vi "creat Output Task.vi"(7 "Configuration":T1={"DAQmxChannel myVolt"={"DAQmxChannel myVinput1"={"PhysicalChanName"="myDAQ2/ai1", "AI_Voltage_Units"=10348, "AI_Max"=5.0, "AI_Min"=-5.0}, "DAQmxChannel myVinput2"={"PhysicalChanName"="", "AI_Voltage_Units"=10348, "AI_Max"=5.0, "AI_Min"=-5.0}, "DAQmxChannel myVoutput1"={"PhysicalChanName"="", "AI_Min"=-5.0, "AI_Max"=5.0, "AI_Voltage_Units"=10348}, "DAQmxChannel myVoutput2"={"PhysicalChanName"="", "AI_Min"=-5.0, "AI_Max"=5.0, "AI_Voltage_Units"=10348}, "Saidmple Clock Input"={"rate"=1000.0, "samples per channel"=100}, "Saidmple Clock Output"={"rate"=1000.0, "samples per channel"=100}}, "Dev"=""} {"DAQmxChannel myVolt"."DAQmxChannel myVoutput2"."AI_Voltage_Units" items=["伏特"=10348, "来自自定义换算"=10065]; "DAQmxChannel myVolt"."DAQmxChannel myVoutput1"."AI_Voltage_Units" items=["伏特"=10348, "来自自定义换算"=10065]; "DAQmxChannel myVolt"."DAQmxChannel myVinput1"."AI_Voltage_Units" items=["伏特"=10348, "来自自定义换算"=10065]; "DAQmxChannel myVolt"."DAQmxChannel myVinput2"."AI_Voltage_Units" items=["伏特"=10348, "来自自定义换算"=10065]}, 11 "Task":refnum<k21>) -> (3 "引用句柄输出":refnum<k21>)   [LabVIEW 2016]
uses:
  Contral/Coniguration.ctl
  <vilib>/DAQmx/create/channels.llb/DAQmx Create Channel (AO-Voltage-Basic).vi
  <vilib>/DAQmx/configure/timing.llb/DAQmx Timing (Sample Clock).vi
panel:
  in  "error in":errorcluster caption="错误输入"
  out "error out":errorcluster caption="错误输出"
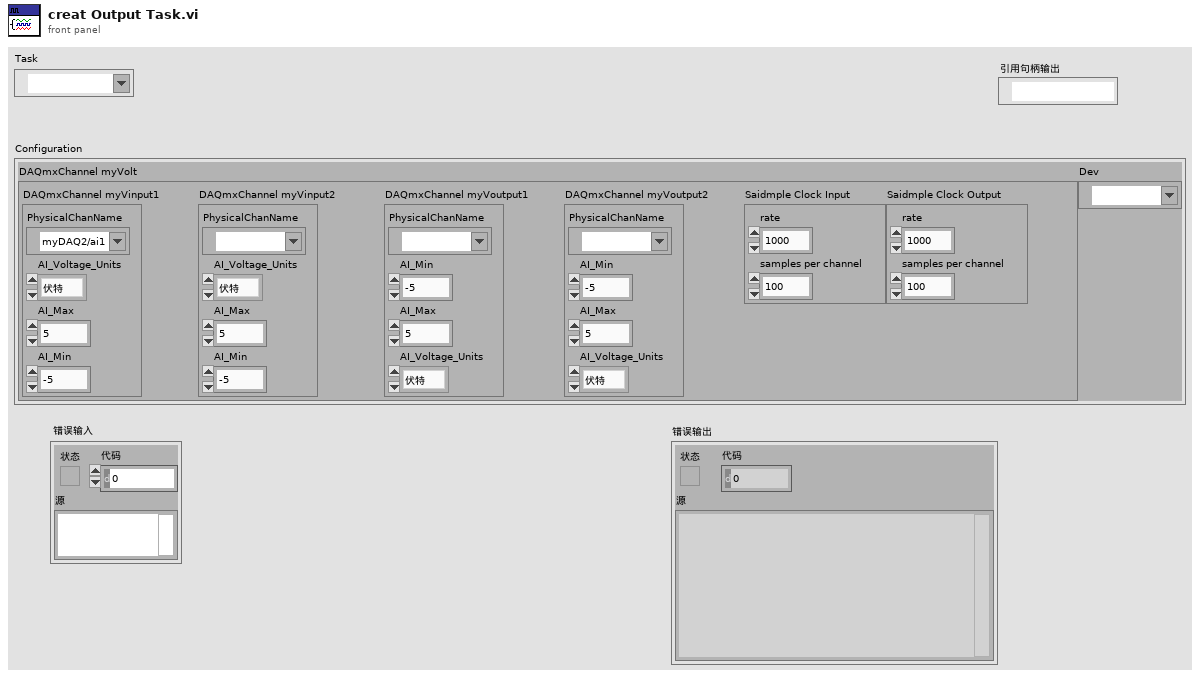
[diagram p1: front panel]
types:
  T1 = typedef "Coniguration.ctl" = cluster{"DAQmxChannel myVolt":cluster{"DAQmxChannel myVinput1":cluster{"PhysicalChanName":tag, "AI_Voltage_Units":i32, "AI_Max":dbl, "AI_Min":dbl}, "DAQmxChannel myVinput2":cluster{"PhysicalChanName":tag, "AI_Voltage_Units":i32, "AI_Max":dbl, "AI_Min":dbl}, "DAQmxChannel myVoutput1":cluster{"PhysicalChanName":tag, "AI_Min":dbl, "AI_Max":dbl, "AI_Voltage_Units":i32}, "DAQmxChannel myVoutput2":cluster{"PhysicalChanName":tag, "AI_Min":dbl, "AI_Max":dbl, "AI_Voltage_Units":i32}, "Saidmple Clock Input":cluster{"rate":dbl, "samples per channel":i32}, "Saidmple Clock Output":cluster{"rate":dbl, "samples per channel":i32}}, "Dev":tag}
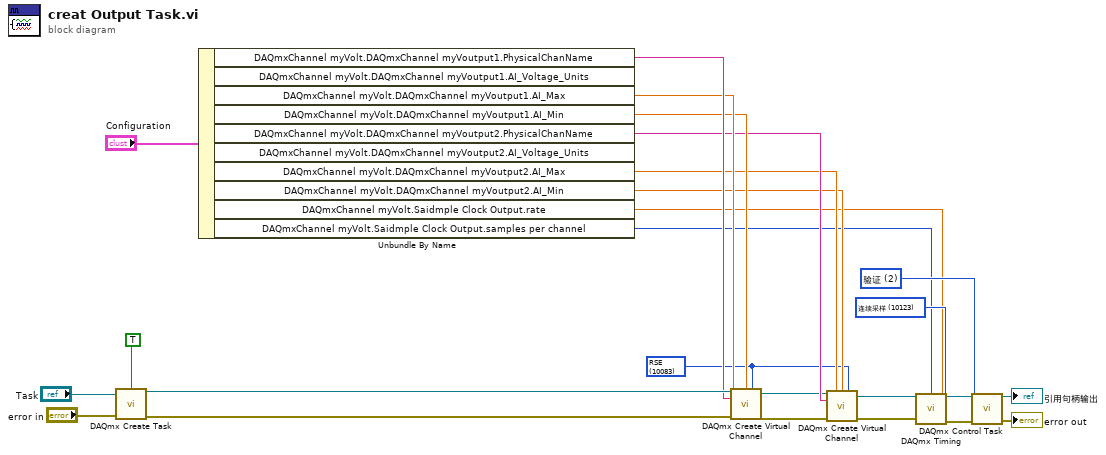
[diagram p0: block diagram]
diagram:
  w19 = 2 items=["验证"=2, "保留"=4, "提交"=3, "未保留"=5, "中止"=6] ("action")
  w22 = 10123 items=["有限采样"=10178, "连续采样"=10123, "硬件定时单点"=12522] ("sample mode")
  w7 = 10083 items=["默认"=-1, "RSE"=10083, "NRSE"=10078, "差分"=10106, "伪差分"=12529] ("input terminal configuration")
  n1 = call <vilib>:"DAQmx Create Task.vi"("auto cleanup"=TRUE, "task to copy"="Task", "error in"="error in") -> ("task out"=w23:refnum<k21>, "error out"=w25:errorcluster)  [unwired: 11 in]
  n2 = Unbundle By Name("Configuration") -> ("DAQmxChannel myVolt.DAQmxChannel myVoutput1.PhysicalChanName"=w17:tag, "DAQmxChannel myVolt.DAQmxChannel myVoutput1.AI_Max"=w16:dbl, "DAQmxChannel myVolt.DAQmxChannel myVoutput1.AI_Min"=w15:dbl, "DAQmxChannel myVolt.DAQmxChannel myVoutput2.PhysicalChanName"=w14:tag, "DAQmxChannel myVolt.DAQmxChannel myVoutput2.AI_Max"=w12:dbl, "DAQmxChannel myVolt.DAQmxChannel myVoutput2.AI_Min"=w11:dbl, "DAQmxChannel myVolt.Saidmple Clock Output.rate"=w2:dbl, "DAQmxChannel myVolt.Saidmple Clock Output.samples per channel"=w1:i32)  [unwired: 2 out]
  n3 = call-poly <vilib>:"DAQmx Create Virtual Channel.vi"("task in"=w23, "maximum value"=w16, "minimum value"=w15, "output terminal configuration"=w7, "physical channels"=w17, "error in"=w25) -> ("task out"=w13:refnum<k21>, "error out"=w10:errorcluster)  [unwired: 8 in]
  n4 = call-poly <vilib>:"DAQmx Create Virtual Channel.vi"("task in"=w13, "maximum value"=w12, "minimum value"=w11, "output terminal configuration"=w7, "physical channels"=w14, "error in"=w10) -> ("task out"=w6:refnum<k21>, "error out"=w5:errorcluster)  [unwired: 8 in]
  n5 = call-poly <vilib>:"DAQmx Timing.vi"("task/channels in"=w6, "sample mode"=w22, "samples per channel"=w1, "rate"=w2, "error in"=w5) -> ("task out"=w21:refnum<k21>, "error out"=w20:errorcluster)  [unwired: 9 in]
  n6 = call <vilib>:"DAQmx Control Task.vi"("task/channels in"=w21, "action"=w19, "error in"=w20) -> ("task out"=→"引用句柄输出":refnum<k21>, "error out"=→"error out":errorcluster)  [unwired: 11 in]
